vi "Audio Solution.vi"() -> ()   [LabVIEW 2013]
uses:
  <vilib>/DAQmx/write.llb/DAQmx Write (Analog 1D Wfm NChan NSamp).vi
  <vilib>/DAQmx/read.llb/DAQmx Read (Analog 1D Wfm NChan NSamp).vi
  <vilib>/DAQmx/create/channels.llb/DAQmx Create Channel (AI-Voltage-Basic).vi
  <vilib>/DAQmx/configure/timing.llb/DAQmx Timing (Sample Clock).vi
  <vilib>/DAQmx/create/channels.llb/DAQmx Create Channel (AO-Voltage-Basic).vi
  <vilib>/DAQmx/miscellaneous.llb/DAQmx Fill In Error Info.vi
  <vilib>/measure/NI_MABase.lvlib
  <resource>/objmgr/daqmx.rc
panel:
  in  "Treble":dbl(slide) scale=0.0..1.0
  in  "Mid-tone":dbl(slide) scale=0.0..1.0
  in  "Bass":dbl(slide) scale=0.0..1.0
  out "frequency":cluster{"f0":dbl, "df":dbl, "magnitude":dbl[]}[](graph)
  in  "Stop Button":bool
  out "data":waveform(dbl)[](graph)
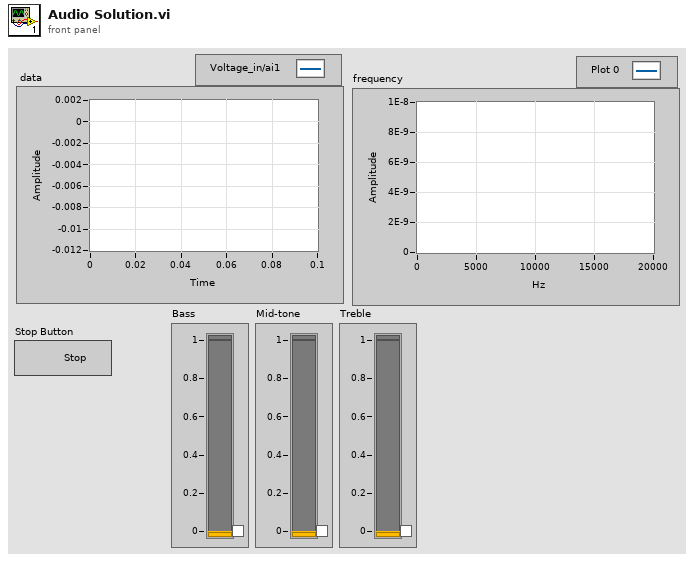
[diagram p1: front panel]
types:
  T1 = enum16{"Sine Wave", "Triangle Wave", "Square Wave", "Sawtooth Wave"}
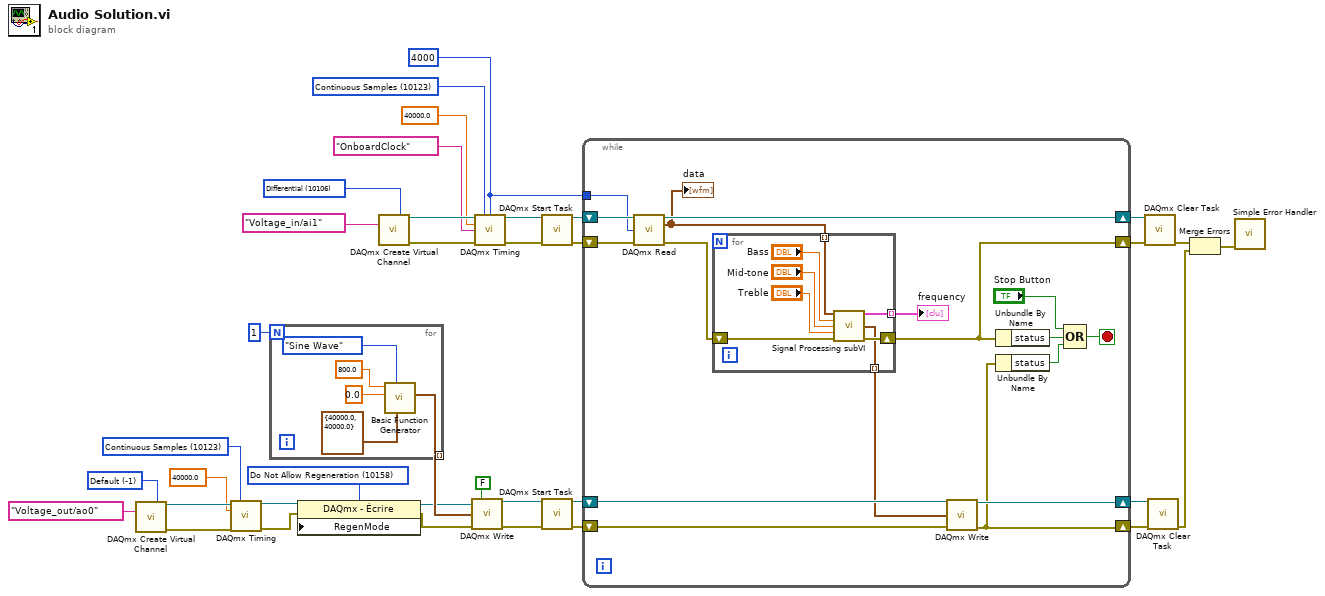
[diagram p0: block diagram]
diagram:
  w5 = 10158 items=["Allow Regeneration"=10097, "Do Not Allow Regeneration"=10158] ("RegenMode")
  w19 = -1 items=["Default"=-1, "RSE"=10083, "Differential"=10106, "Pseudodifferential"=12529] ("output terminal configuration")
  w21 = 10123 items=["Finite Samples"=10178, "Continuous Samples"=10123, "Hardware Timed Single Point"=12522] ("sample mode")
  w24 = 4000 ("samples per channel")
  w31 = 10123 items=["Finite Samples"=10178, "Continuous Samples"=10123, "Hardware Timed Single Point"=12522] ("sample mode")
  w36 = 10106 items=["default"=-1, "RSE"=10083, "NRSE"=10078, "Differential"=10106, "Pseudodifferential"=12529] ("input terminal configuration")
  n1 = call-poly <vilib>:"DAQmx Create Virtual Channel.vi"("output terminal configuration"=w19, "physical channels"=tag "Voltage_out/ao0") -> ("task out"=w23:refnum<k21>, "error out"=w22:errorcluster)  [unwired: 12 in]
  n2 = call-poly <vilib>:"DAQmx Timing.vi"("task/channels in"=w23, "sample mode"=w21, "rate"=40000.0, "error in"=w22) -> ("task out"=w9:refnum<k21>, "error out"=w8:errorcluster)  [unwired: 10 in]
  n3 = for {
    N: 1 -> [_]
    tunnel: [w38] -> w15 mode=indexing
    n4 = call <vilib>:"Basic Function Generator.vi"("sampling info"=cluster{"Fs":dbl, "#s":dbl} {"Fs"=40000.0, "#s"=40000.0}, "signal type"=T1."Sine Wave", "amplitude"=0.0, "frequency"=800.0) -> ("signal out"=w38:waveform(dbl))  [unwired: 5 in, 2 out]
  }
  n5 = property class="DAQmx - Écrire"(reference=w9, error in=w8, "RegenMode"=w5) -> (reference out=w7:refnum<k21>, error out=w6:errorcluster)
  n6 = call-poly <vilib>:"DAQmx Create Virtual Channel.vi"("input terminal configuration"=w36, "physical channels"=tag "Voltage_in/ai1") -> ("task out"=w35:refnum<k21>, "error out"=w34:errorcluster)  [unwired: 12 in]
  n7 = call-poly <vilib>:"DAQmx Write.vi"("task/channels in"=w7, "auto start"=FALSE, "data"=w15, "error in"=w6) -> ("task out"=w16:refnum<k21>, "error out"=w17:errorcluster)  [unwired: 9 in, 1 out]
  n8 = call-poly <vilib>:"DAQmx Timing.vi"("task/channels in"=w35, "sample mode"=w31, "samples per channel"=w24, "rate"=40000.0, "source"=tag "OnboardClock", "error in"=w34) -> ("task out"=w30:refnum<k21>, "error out"=w29:errorcluster)  [unwired: 8 in]
  n9 = call <vilib>:"DAQmx Start Task.vi"("task/channels in"=w30, "error in"=w29) -> ("task out"=w25:refnum<k21>, "error out"=w28:errorcluster)  [unwired: 12 in]
  n10 = call <vilib>:"DAQmx Start Task.vi"("task/channels in"=w16, "error in"=w17) -> ("task out"=w14:refnum<k21>, "error out"=w11:errorcluster)  [unwired: 12 in]
  n11 = while {
    tunnel: w24 -> [w55]
    shift-right: [w52] -> w12
    shift-left: w11 -> [w51]
    shift-right: [w53] -> w13
    shift-left: w14 -> [w54]
    shift-right: [w57] -> w26
    shift-left: w28 -> [w59]
    shift-right: [w58] -> w27
    shift-left: w25 -> [w56]
    stop <- w44 stop-if-true
    n12 = call-poly <vilib>:"DAQmx Read.vi"("task/channels in"=w56, "number of samples per channel"=w55, "error in"=w59) -> ("task out"=w58:refnum<k21>, "data"=w47:waveform(dbl)[], "error out"=w48:errorcluster)  [unwired: 10 in]
    "data" <- w47
    n13 = for {
      tunnel: [w66] -> w49 mode=indexing
      tunnel: w47 -> [w64] mode=indexing
      tunnel: [w60] -> w43 mode=indexing
      shift-right: [w67] -> w57
      shift-left: w48 -> [w65]
      n14 = call "Signal Processing subVI.vi"("data"=w64, "Bass"="Bass", "Mid-tone"="Mid-tone", "Treble"="Treble", "error in (no error)"=w65) -> ("Power Spectrum / PSD"=w66:cluster{"f0":dbl, "df":dbl, "magnitude":dbl[]}, "output waveform"=w60:waveform(dbl), "error out"=w67:errorcluster)  [unwired: 8 in]
    }
    "frequency" <- w49
    n15 = call-poly <vilib>:"DAQmx Write.vi"("task/channels in"=w54, "data"=w43, "error in"=w51) -> ("task out"=w53:refnum<k21>, "error out"=w52:errorcluster)  [unwired: 10 in, 1 out]
    n16 = Unbundle By Name(w57) -> ("status"=w50:bool)
    n17 = Unbundle By Name(w52) -> ("status"=w45:bool)
    n18 = Compound Arithmetic op=OR("Stop Button", w50, w45) -> (w44:bool)
  }
  n19 = call <vilib>:"DAQmx Clear Task.vi"("task in"=w27, "error in"=w26) -> ("error out"=w4:errorcluster)  [unwired: 13 in]
  n20 = call <vilib>:"DAQmx Clear Task.vi"("task in"=w13, "error in"=w12) -> ("error out"=w3:errorcluster)  [unwired: 13 in]
  n21 = Merge Errors(w4, w3) -> (w2:errorcluster)
  n22 = call <vilib>:"Simple Error Handler.vi"("error in (no error)"=w2) -> ()  [unwired: 4 in, 5 out]
